vi "Initialize Routing Channel Page (State Configuration).vi"(8 "error in (no error)":errorcluster, 10 "Routing Channel Page Controls":T1, 11 "Routing Channel Ref in":T2 format="%.0x") -> (0 "error out":errorcluster, 3 "Routing Channel Ref out":T2 format="%.0x")   [LabVIEW 2017, in "Routing and Faulting System Explorer.lvlib"]
uses:
  Routing and Faulting System Explorer.lvlib
  <vilib>/NI Veristand/Custom Device API/Custom Device Item Ref.ctl
  Routing Channel Page Controls.ctl
  Routing Channel Initial Tab.ctl
  Routing Channel Configuration Tab.ctl
  Shared/Constants.vi
  Scripting/Routing and Faulting Scripting.lvlib
  Shared/Routing and Faulting Shared.lvlib
  <vilib>/NI VeriStand/Custom Device API/Custom Device API.lvlib
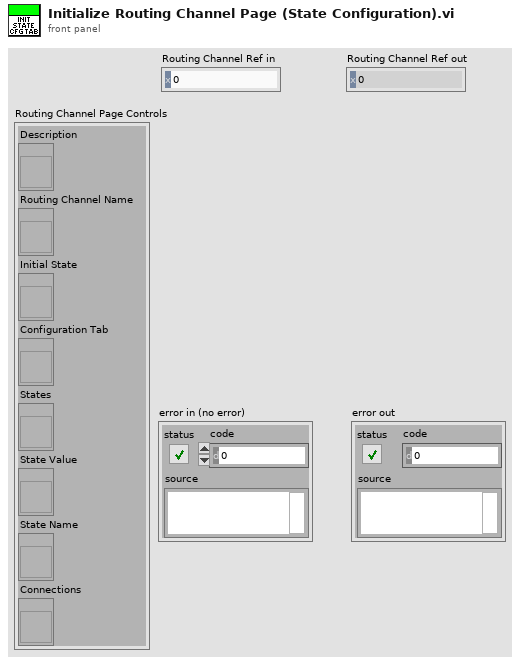
[diagram p1: front panel]
types:
  T1 = typedef "Routing and Faulting System Explorer.lvlib/Routing Channel Page Controls.ctl" = cluster{"Description":refnum<vi>, "Routing Channel Name":refnum<vi>, "Initial State":refnum<vi>, "Configuration Tab":refnum<vi>, "States":refnum<vi>, "State Value":refnum<vi>, "State Name":refnum<vi>, "Connections":refnum<vi>}
  T2 = typedef "Custom Device API.lvlib/Custom Device Item Ref.ctl" = u64
  T3 = typedef "Routing and Faulting System Explorer.lvlib/Routing Channel Initial Tab.ctl" = enum16{"Route Configuration", "State Configuration", "State Conf if Empty"}
  T4 = enum8{"Enabled", "Disabled", "Disabled and Grayed Out"}
  T5 = typedef "Routing and Faulting System Explorer.lvlib/Routing Channel Configuration Tab.ctl" = enum32{"Route Configuation", "State Configuration"}
  T6 = typedef "Routing and Faulting System Explorer.lvlib/State-Value Row.ctl" = cluster{"State":T7, "State Value":string}
  T7 = typedef "Routing and Faulting System Explorer.lvlib/State Control.ctl" = string
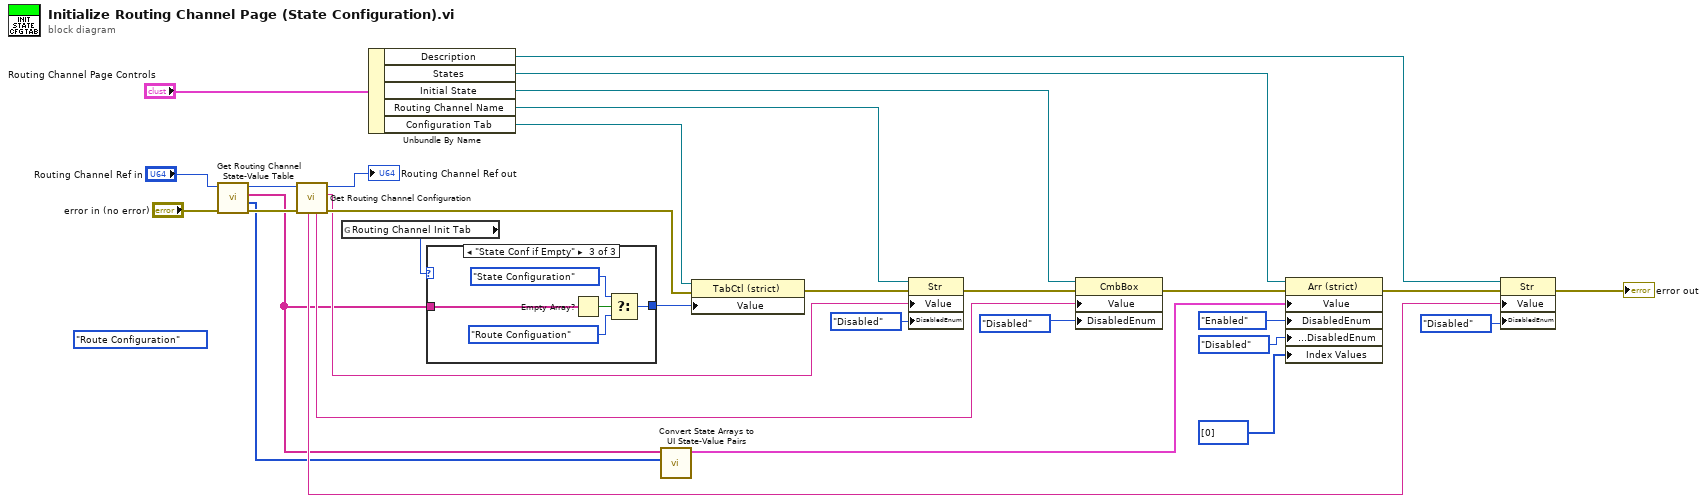
[diagram p0: block diagram]
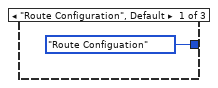
[diagram p2: hidden frame]
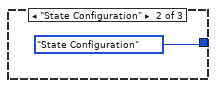
[diagram p3: hidden frame]
diagram:
  (unwired) Routing_Channel_Initial_Tab."Route Configuration"
  n1 = call "Get Routing Channel State-Value Table.vi"("error in (no error)"="error in (no error)", "Channel Ref in"="Routing Channel Ref in") -> ("error out"=w22:errorcluster, "State Values"=w15:i32[], "State Names"=w2:string[], "Channel Ref out"=w23:T2)  [unwired: 6 in]
  n2 = call "Get Routing Channel Configuration.vi"("error in (no error)"=w22, "Channel Ref in"=w23) -> ("error out"=w20:errorcluster, "Channel Name"=w19:string, "Channel Ref out"=→"Routing Channel Ref out":T2, "Initial State"=w8:string, "Description"=w29:string)  [unwired: 4 in, 1 out]
  n3 = global read "Constants.vi" "Routing Channel Init Tab"() -> (w1:T3)
  n4 = Unbundle By Name("Routing Channel Page Controls") -> ("Description"=w28:refnum<vi>, "States"=w17:refnum<vi>, "Initial State"=w24:refnum<vi>, "Routing Channel Name"=w25:refnum<vi>, "Configuration Tab"=w27:refnum<vi>)
  n5 = case shown="\"State Conf if Empty\"" w1 {
    tunnel: [Routing_Channel_Configuration_Tab."Route Configuation" ("Routing Channel Configuration Tab") Routing_Channel_Configuration_Tab."State Configuration" ("Routing Channel Configuration Tab") w35] -> w26
    tunnel: w2 -> [_ _ w34]
    frame "Route Configuration", Default {
    }
    frame "State Configuration" {
    }
    frame "State Conf if Empty" {
      n6 = Empty Array?(array=w34) -> (empty?=w36:bool)
      n7 = Select(t=Routing_Channel_Configuration_Tab."State Configuration" ("Routing Channel Configuration Tab"), s=w36, f=Routing_Channel_Configuration_Tab."Route Configuation" ("Routing Channel Configuration Tab")) -> (s? t:f=w35:T5)
    }
  }
  n8 = call "Convert State Arrays to UI State-Value Pairs.vi"("State Values"=w15, "State Names"=w2) -> ("State-Value Pairs"=w11:T6[])  [unwired: 9 in]
  n9 = property class="TabCtl (strict)"(reference=w27, error in=w20, "Value"=w26) -> (error out=w21:errorcluster)  [unwired: 1 out]
  n10 = property class="Str"(reference=w25, error in=w21, "Value"=w19, "DisabledEnum"=T4."Disabled" ("Array Element.Disabled")) -> (error out=w30:errorcluster)  [unwired: 1 out]
  n11 = property class="CmbBox"(reference=w24, error in=w30, "Value"=w8, "DisabledEnum"=T4."Disabled" ("Array Element.Disabled")) -> (error out=w18:errorcluster)  [unwired: 1 out]
  n12 = property class="Arr (strict)"(reference=w17, error in=w18, "Value"=w11, "DisabledEnum"=T4."Enabled" ("Disabled"), "Array Element.DisabledEnum"=T4."Disabled" ("Array Element.Disabled"), "Index Values"=u32[] [0]) -> (error out=w16:errorcluster)  [unwired: 1 out]
  n13 = property class="Str"(reference=w28, error in=w16, "Value"=w29, "DisabledEnum"=T4."Disabled" ("Array Element.Disabled")) -> (error out=→"error out":errorcluster)  [unwired: 1 out]
